vi "initiateProducts.vi"(0 "reference in":refnum<class "Project Panels.lvclass">, 5 "error in (no error)":errorcluster) -> (14 "reference out":refnum<class "Project Panels.lvclass">, 16 "tables":T1, 19 "error out":errorcluster)   [LabVIEW 2016, in "Project Panels.lvclass"]
uses:
  Project Panels.lvclass
  SYS/Devices Controller_llb/Devices Controller.lvclass
  APP/k4b2_class/k4b2.lvclass
  APP/rmr_class/rmr.lvclass
  APP/bodpod_class/bodpod.lvclass
  APP/cpet_class/cpet.lvclass
  APP/fitmate_class/fitmate.lvclass
  APP/peapod_class/peapod.lvclass
  APP/k5_class/k5.lvclass
  APP/bb-pft_class/bb-pft.lvclass
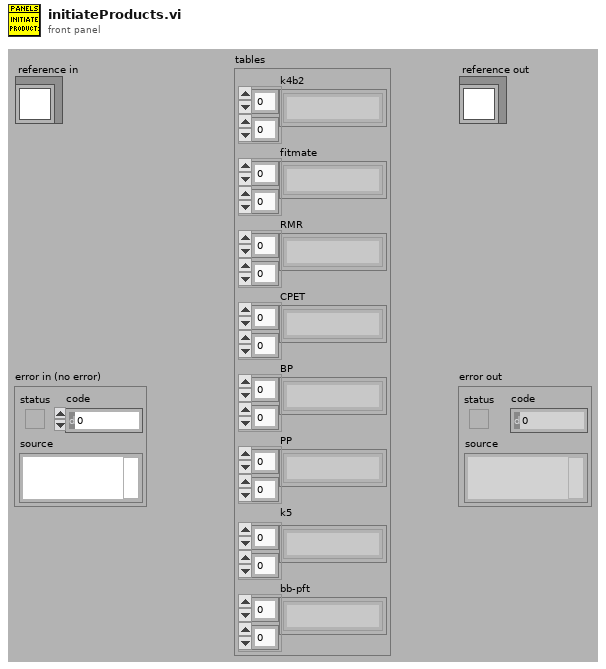
[diagram p1: front panel]
types:
  T1 = cluster{"k4b2":string[][], "fitmate":string[][], "RMR":string[][], "CPET":string[][], "BP":string[][], "PP":string[][], "k5":string[][], "bb-pft":string[][]}
  T2 = typedef "Project Panels.lvclass/ObjectAttributesRef.ctl" = refnum<data-value>
  T3 = typedef "Project Panels.lvclass/ObjectAttributes.ctl" = cluster{"MyAttribute":dbl, "device_controller_ref":refnum<class "Devices Controller.lvclass">, "file_controller_ref":refnum<class "File Controller.lvclass">, "item_controller_ref":refnum<class "Items Controller.lvclass">, "item_tables":cluster{"checkIN":string[][], "checkOUT":string[][], "storage":string[][]}, "quickbook_table":cluster{"notes":string[][]}, "notification_controller_ref":refnum<class "Notification Controller.lvclass">, "partstracking_controller_ref":refnum<class "PartsTracking Controller.lvclass">, "product_tables":cluster{"k4b2":string[][], "fitmate":string[][], "RMR":string[][], "CPET":string[][], "BP":string[][], "PP":string[][], "k5":string[][], "bb-pft":string[][]}, "rowsColour":u32[], "low_resolution?":bool, "run_python?":bool}
  T4 = cluster{"k4b2_refs":refnum<class "k4b2.lvclass">[], "rmr_refs":refnum<class "rmr.lvclass">[], "bod_pod_refs":refnum<class "bodpod.lvclass">[], "cpet_refs":refnum<class "cpet.lvclass">[], "fitmate_refs":refnum<class "fitmate.lvclass">[], "pea_pod_refs":refnum<class "peapod.lvclass">[], "k5_refs":refnum<class "k5.lvclass">[], "bb-pft_refs":refnum<class "bb-pft.lvclass">[]}
  T5 = typedef "Devices Controller.lvclass/deviceType.ctl" = enum16{"k5", "k4b2", "fitmate", "cpet", "rmr", "bodyBoxPft", "bp", "pp"}
  T6 = cluster{"deviceType":T5, "S/N":string, "SW":string, "Description":string, "Account":string, "System's Location":string, "End User":string, "Email":string, "City":string, "LastChange":string, "Service By":string, "Exp Date":string, "FollowUp Sent":string, "FollowUp Accepted":string, "Note":string}
  T7 = cluster{"deviceType":T5, "S/N":string, "SW":string, "Description":string, "Account":string, "System's Location":string, "End User":string, "Email":string, "City":string, "FollowUp Sent":string, "FollowUp Accepted":string, "Note":string}
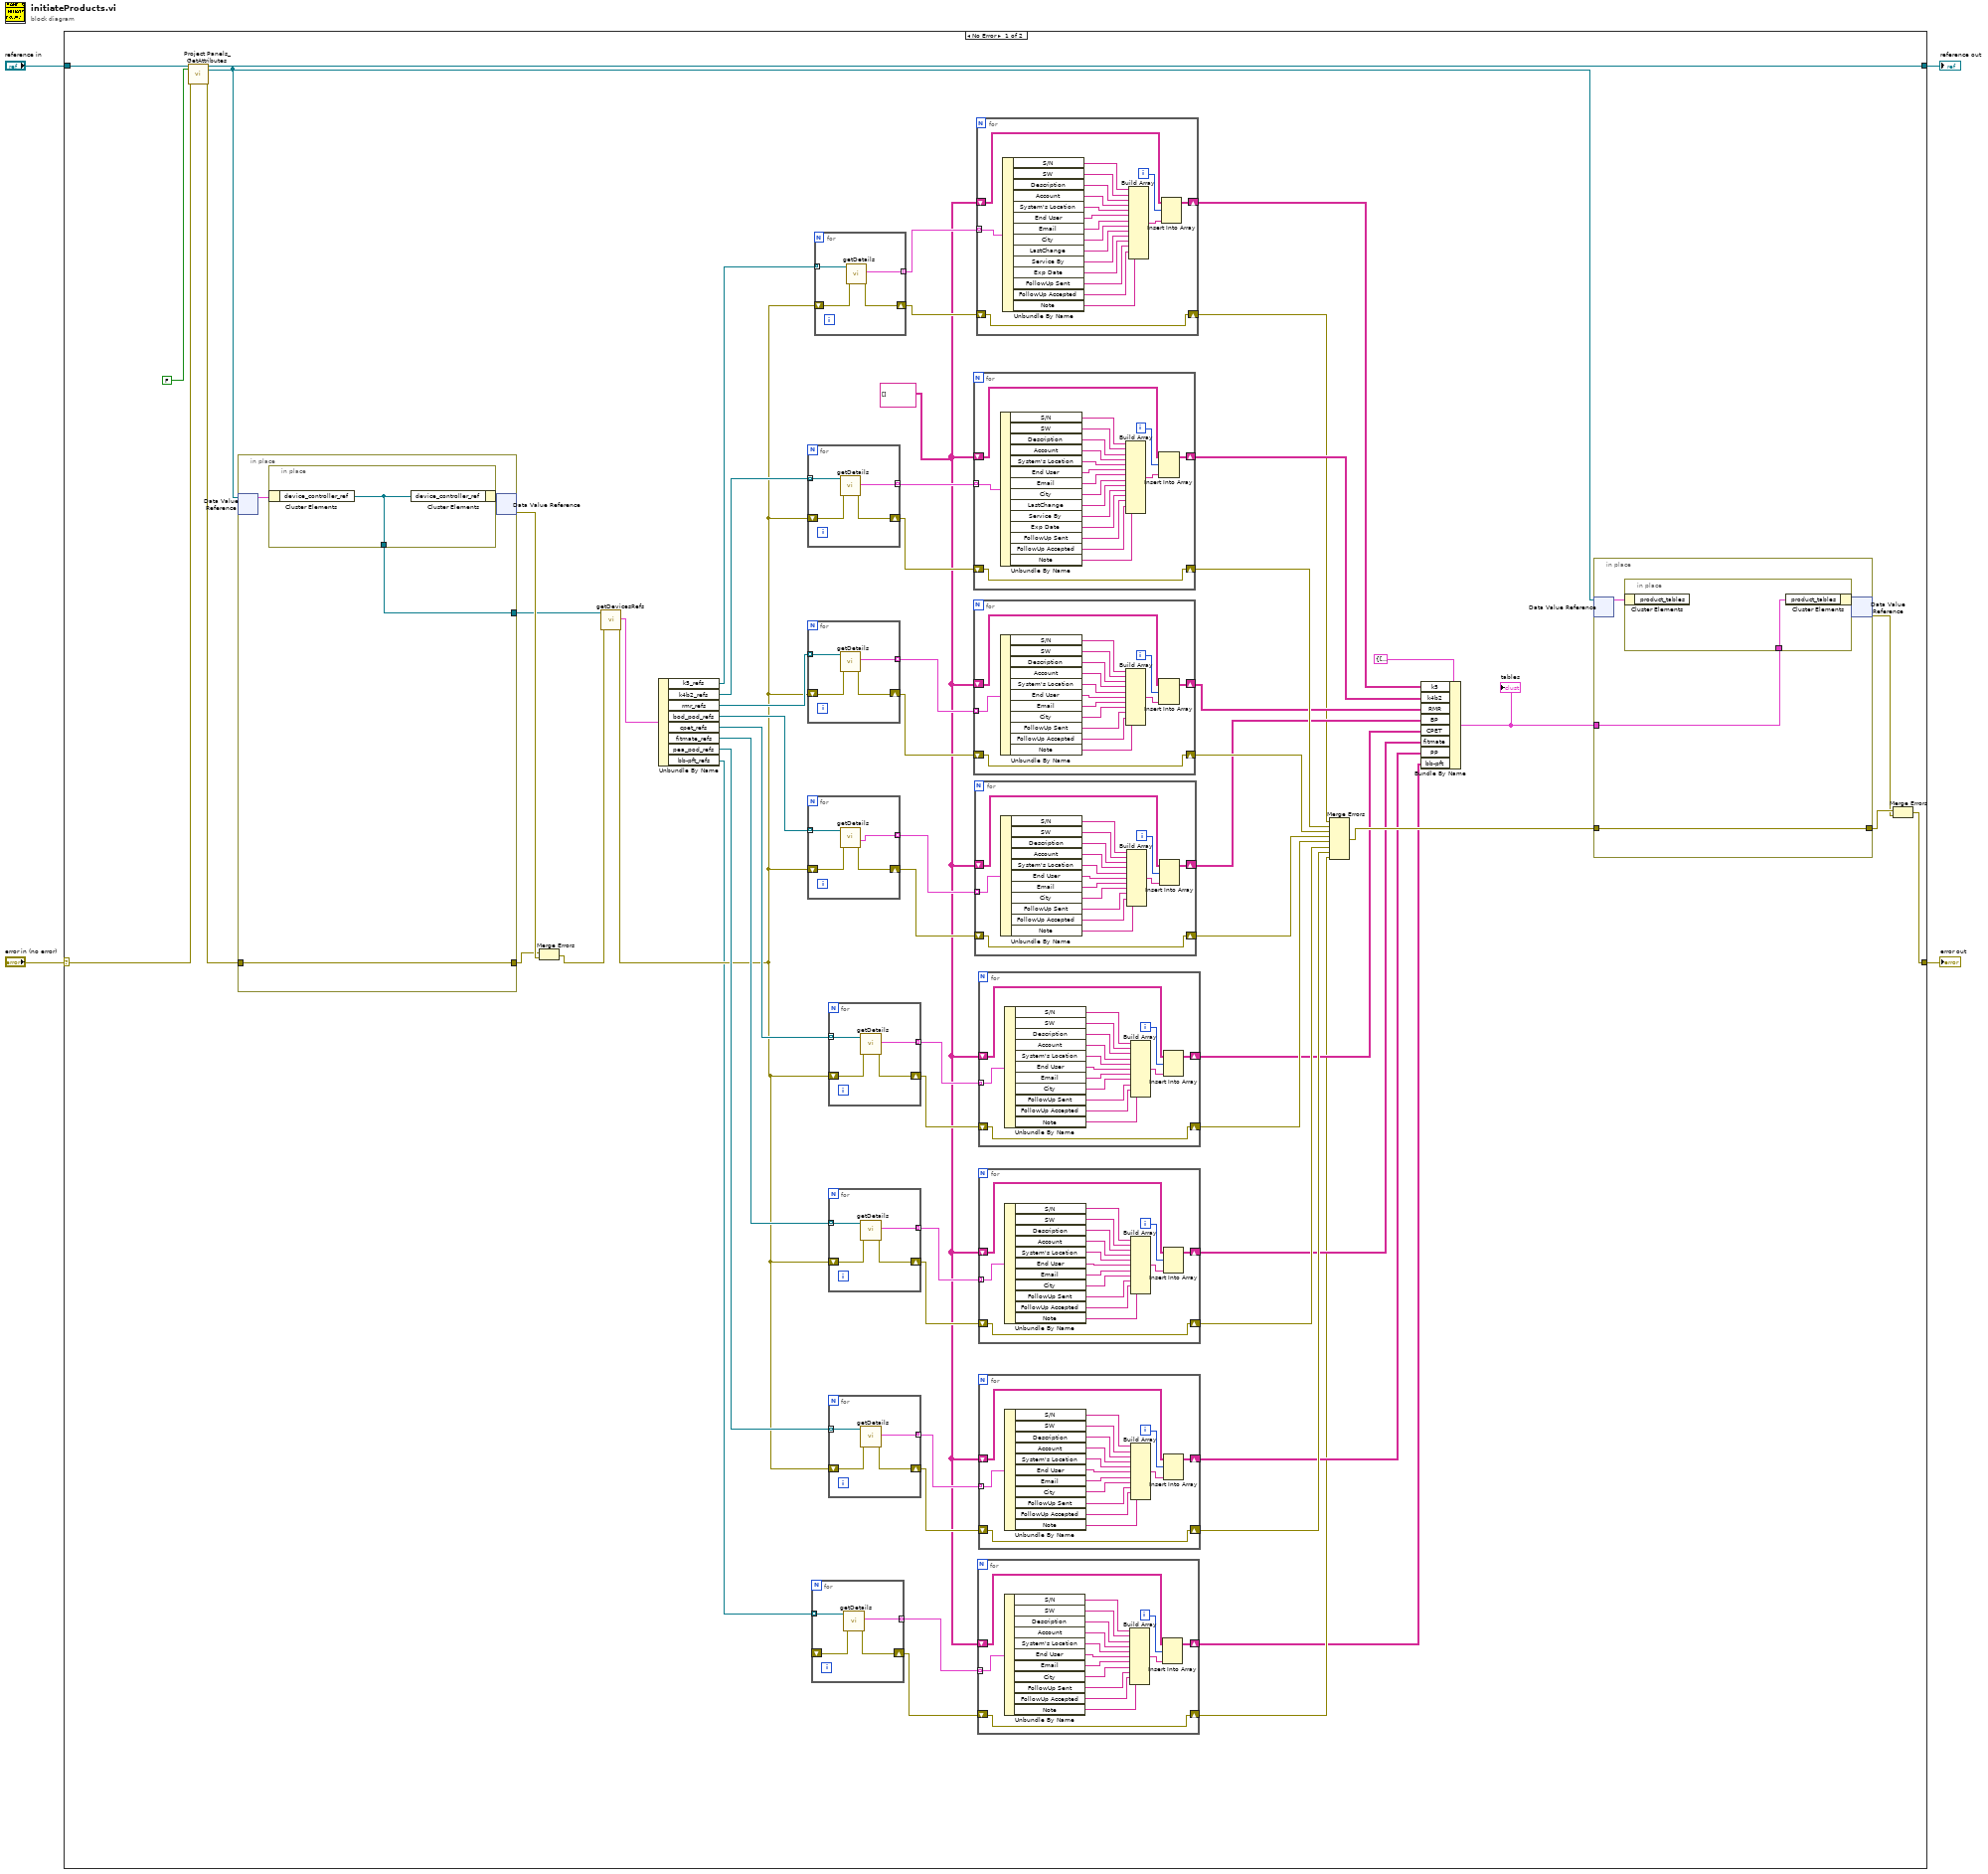
[diagram p0: block diagram]
diagram:
  n1 = case shown="No Error" "error in (no error)" {
    selector: "error in (no error)" -> [w20 w249]
    tunnel: [w21 w249] -> w3
    tunnel: [w58 w248] -> w1
    tunnel: "reference in" -> [w61 w248]
    frame No Error {
      w10 = string[][] [] ("Table Control")
      n2 = call "Project Panels_GetAttributes.vi"("reference in"=w61, "return data? (T)"=FALSE, "error in (no error)"=w20) -> ("reference out"=w58:refnum<class "Project Panels.lvclass">, "attributes ref"=w31:T2, "error out"=w59:errorcluster)  [unwired: 13 in, 1 out]
      n3 = in-place {
        in-place-border: w59 -> [w244]
        in-place-border: [w244] -> w62
        in-place-border: [w243] -> w19
        n4 = in-place-dvr #1(w31) -> (w245:T3)  [unwired: 1 out]
        n5 = in-place {
          in-place-border: [w247] -> w243
          n6 = in-place-cluster #2(w245) -> ("device_controller_ref"=w247:refnum<class "Devices Controller.lvclass">)
          n7 = in-place-cluster #2("device_controller_ref"=w247) -> (w246:T3)
        }
        n8 = in-place-dvr #1(w246) -> (w63:errorcluster)  [unwired: 1 out]
      }
      n9 = Merge Errors(w62, w63) -> (w56:errorcluster)
      n10 = call "getDevicesRefs.vi"("error in (no error)"=w56, "reference in"=w19) -> ("error out"=w14:errorcluster, "devices_refs"=w57:T4)  [unwired: 7 in, 1 out]
      n11 = Unbundle By Name(w57) -> ("k5_refs"=w15:refnum<class "k5.lvclass">[], "k4b2_refs"=w55:refnum<class "k4b2.lvclass">[], "rmr_refs"=w53:refnum<class "rmr.lvclass">[], "bod_pod_refs"=w51:refnum<class "bodpod.lvclass">[], "cpet_refs"=w47:refnum<class "cpet.lvclass">[], "fitmate_refs"=w44:refnum<class "fitmate.lvclass">[], "pea_pod_refs"=w41:refnum<class "peapod.lvclass">[], "bb-pft_refs"=w8:refnum<class "bb-pft.lvclass">[])
      n12 = for {
        shift-right: [w241] -> w17
        shift-left: w14 -> [w242]
        tunnel: [w240] -> w54 mode=indexing
        tunnel: w55 -> [w239] mode=indexing
        n13 = call "getDetails.vi"("error in (no error)"=w242, "reference in"=w239) -> ("error out"=w241:errorcluster, "details"=w240:T6)  [unwired: 7 in, 1 out]
      }
      n14 = for {
        shift-right: [w217] -> w52
        shift-left: w14 -> [w218]
        tunnel: [w216] -> w49 mode=indexing
        tunnel: w53 -> [w215] mode=indexing
        n15 = call "getDetails.vi"("error in (no error)"=w218, "reference in"=w215) -> ("error out"=w217:errorcluster, "details"=w216:T7)  [unwired: 7 in, 1 out]
      }
      n16 = for {
        shift-right: [w179] -> w48
        shift-left: w14 -> [w180]
        tunnel: [w177] -> w50 mode=indexing
        tunnel: w51 -> [w178] mode=indexing
        n17 = call "getDetails.vi"("error in (no error)"=w180, "reference in"=w178) -> ("error out"=w179:errorcluster, "details"=w177:T7)  [unwired: 7 in, 1 out]
      }
      n18 = for {
        shift-right: [w83] -> w11
        shift-left: _ -> [w84]
        tunnel: [w82] -> w9 mode=indexing
        tunnel: w8 -> [w81] mode=indexing
        n19 = call "getDetails.vi"("error in (no error)"=w84, "reference in"=w81) -> ("error out"=w83:errorcluster, "details"=w82:T7)  [unwired: 7 in, 1 out]
      }
      n20 = for {
        shift-right: [w87] -> w16
        shift-left: w14 -> [w88]
        tunnel: [w86] -> w13 mode=indexing
        tunnel: w15 -> [w85] mode=indexing
        n21 = call "getDetails.vi"("error in (no error)"=w88, "reference in"=w85) -> ("error out"=w87:errorcluster, "details"=w86:T6)  [unwired: 7 in, 1 out]
      }
      n22 = for {
        shift-right: [w158] -> w45
        shift-left: w14 -> [w159]
        tunnel: [w156] -> w46 mode=indexing
        tunnel: w47 -> [w157] mode=indexing
        n23 = call "getDetails.vi"("error in (no error)"=w159, "reference in"=w157) -> ("error out"=w158:errorcluster, "details"=w156:T7)  [unwired: 7 in, 1 out]
      }
      n24 = for {
        shift-right: [w137] -> w43
        shift-left: w14 -> [w138]
        tunnel: [w136] -> w42 mode=indexing
        tunnel: w44 -> [w135] mode=indexing
        n25 = call "getDetails.vi"("error in (no error)"=w138, "reference in"=w135) -> ("error out"=w137:errorcluster, "details"=w136:T7)  [unwired: 7 in, 1 out]
      }
      n26 = for {
        shift-right: [w116] -> w40
        shift-left: w14 -> [w117]
        tunnel: [w115] -> w39 mode=indexing
        tunnel: w41 -> [w114] mode=indexing
        n27 = call "getDetails.vi"("error in (no error)"=w117, "reference in"=w114) -> ("error out"=w116:errorcluster, "details"=w115:T7)  [unwired: 7 in, 1 out]
      }
      n28 = for {
        tunnel: w54 -> [w236] mode=indexing
        shift-right: [w237] -> w30
        shift-left: w10 -> [w238]
        shift-right: [w220] -> w37
        shift-left: w17 -> [w220]
        i -> [w233]
        n29 = Unbundle By Name(w236) -> ("S/N"=w235:string, "SW"=w232:string, "Description"=w231:string, "Account"=w230:string, "System's Location"=w229:string, "End User"=w228:string, "Email"=w227:string, "City"=w226:string, "LastChange"=w225:string, "Service By"=w224:string, "Exp Date"=w223:string, "FollowUp Sent"=w222:string, "FollowUp Accepted"=w221:string, "Note"=w219:string)
        n30 = Build Array(w235, w232, w231, w230, w229, w228, w227, w226, w225, w224, w223, w222, w221, w219) -> (w234:string[])
        n31 = Insert Into Array(array=w238, index (row)=w233, new element=w234) -> (w237:string[][])  [unwired: 1 in]
      }
      n32 = for {
        tunnel: w49 -> [w212] mode=indexing
        shift-right: [w213] -> w28
        shift-left: w10 -> [w214]
        shift-right: [w199] -> w36
        shift-left: w52 -> [w199]
        i -> [w209]
        n33 = Unbundle By Name(w212) -> ("S/N"=w211:string, "SW"=w208:string, "Description"=w207:string, "Account"=w206:string, "System's Location"=w205:string, "End User"=w204:string, "Email"=w203:string, "City"=w202:string, "FollowUp Sent"=w201:string, "FollowUp Accepted"=w200:string, "Note"=w198:string)
        n34 = Build Array(w211, w208, w207, w206, w205, w204, w203, w202, w201, w200, w198) -> (w210:string[])
        n35 = Insert Into Array(array=w214, index (row)=w209, new element=w210) -> (w213:string[][])  [unwired: 1 in]
      }
      n36 = for {
        tunnel: w50 -> [w195] mode=indexing
        shift-right: [w196] -> w27
        shift-left: w10 -> [w197]
        shift-right: [w183] -> w35
        shift-left: w48 -> [w183]
        i -> [w193]
        n37 = Unbundle By Name(w195) -> ("S/N"=w194:string, "SW"=w192:string, "Description"=w191:string, "Account"=w190:string, "System's Location"=w189:string, "End User"=w188:string, "Email"=w187:string, "City"=w186:string, "FollowUp Sent"=w185:string, "FollowUp Accepted"=w184:string, "Note"=w181:string)
        n38 = Build Array(w194, w192, w191, w190, w189, w188, w187, w186, w185, w184, w181) -> (w182:string[])
        n39 = Insert Into Array(array=w197, index (row)=w193, new element=w182) -> (w196:string[][])  [unwired: 1 in]
      }
      n40 = for {
        tunnel: w13 -> [w106] mode=indexing
        shift-right: [w107] -> w12
        shift-left: w10 -> [w108]
        shift-right: [w90] -> w7
        shift-left: w16 -> [w90]
        i -> [w103]
        n41 = Unbundle By Name(w106) -> ("S/N"=w105:string, "SW"=w102:string, "Description"=w101:string, "Account"=w100:string, "System's Location"=w99:string, "End User"=w98:string, "Email"=w97:string, "City"=w96:string, "LastChange"=w95:string, "Service By"=w94:string, "Exp Date"=w93:string, "FollowUp Sent"=w92:string, "FollowUp Accepted"=w91:string, "Note"=w89:string)
        n42 = Build Array(w105, w102, w101, w100, w99, w98, w97, w96, w95, w94, w93, w92, w91, w89) -> (w104:string[])
        n43 = Insert Into Array(array=w108, index (row)=w103, new element=w104) -> (w107:string[][])  [unwired: 1 in]
      }
      n44 = for {
        tunnel: w9 -> [w78] mode=indexing
        shift-right: [w79] -> w5
        shift-left: w10 -> [w80]
        shift-right: [w65] -> w6
        shift-left: w11 -> [w65]
        i -> [w75]
        n45 = Unbundle By Name(w78) -> ("S/N"=w77:string, "SW"=w74:string, "Description"=w73:string, "Account"=w72:string, "System's Location"=w71:string, "End User"=w70:string, "Email"=w69:string, "City"=w68:string, "FollowUp Sent"=w67:string, "FollowUp Accepted"=w66:string, "Note"=w64:string)
        n46 = Build Array(w77, w74, w73, w72, w71, w70, w69, w68, w67, w66, w64) -> (w76:string[])
        n47 = Insert Into Array(array=w80, index (row)=w75, new element=w76) -> (w79:string[][])  [unwired: 1 in]
      }
      n48 = for {
        tunnel: w46 -> [w174] mode=indexing
        shift-right: [w175] -> w26
        shift-left: w10 -> [w176]
        shift-right: [w162] -> w34
        shift-left: w45 -> [w162]
        i -> [w172]
        n49 = Unbundle By Name(w174) -> ("S/N"=w173:string, "SW"=w171:string, "Description"=w170:string, "Account"=w169:string, "System's Location"=w168:string, "End User"=w167:string, "Email"=w166:string, "City"=w165:string, "FollowUp Sent"=w164:string, "FollowUp Accepted"=w163:string, "Note"=w160:string)
        n50 = Build Array(w173, w171, w170, w169, w168, w167, w166, w165, w164, w163, w160) -> (w161:string[])
        n51 = Insert Into Array(array=w176, index (row)=w172, new element=w161) -> (w175:string[][])  [unwired: 1 in]
      }
      n52 = for {
        tunnel: w42 -> [w153] mode=indexing
        shift-right: [w154] -> w25
        shift-left: w10 -> [w155]
        shift-right: [w141] -> w33
        shift-left: w43 -> [w141]
        i -> [w151]
        n53 = Unbundle By Name(w153) -> ("S/N"=w152:string, "SW"=w150:string, "Description"=w149:string, "Account"=w148:string, "System's Location"=w147:string, "End User"=w146:string, "Email"=w145:string, "City"=w144:string, "FollowUp Sent"=w143:string, "FollowUp Accepted"=w142:string, "Note"=w139:string)
        n54 = Build Array(w152, w150, w149, w148, w147, w146, w145, w144, w143, w142, w139) -> (w140:string[])
        n55 = Insert Into Array(array=w155, index (row)=w151, new element=w140) -> (w154:string[][])  [unwired: 1 in]
      }
      n56 = for {
        tunnel: w39 -> [w132] mode=indexing
        shift-right: [w133] -> w24
        shift-left: w10 -> [w134]
        shift-right: [w120] -> w32
        shift-left: w40 -> [w120]
        i -> [w130]
        n57 = Unbundle By Name(w132) -> ("S/N"=w131:string, "SW"=w129:string, "Description"=w128:string, "Account"=w127:string, "System's Location"=w126:string, "End User"=w125:string, "Email"=w124:string, "City"=w123:string, "FollowUp Sent"=w122:string, "FollowUp Accepted"=w121:string, "Note"=w118:string)
        n58 = Build Array(w131, w129, w128, w127, w126, w125, w124, w123, w122, w121, w118) -> (w119:string[])
        n59 = Insert Into Array(array=w134, index (row)=w130, new element=w119) -> (w133:string[][])  [unwired: 1 in]
      }
      n60 = Merge Errors(w7, w37, w36, w35, w34, w33, w32, w6) -> (w38:errorcluster)
      n61 = Bundle By Name(cluster=T1 {"k4b2"=[], "fitmate"=[], "RMR"=[], "CPET"=[], "BP"=[], "PP"=[], "k5"=[], "bb-pft"=[]} ("tables 2"), "k5"=w12, "k4b2"=w30, "RMR"=w28, "BP"=w27, "CPET"=w26, "fitmate"=w25, "PP"=w24, "bb-pft"=w5) -> (w29:T1)
      "tables" <- w29
      n62 = in-place {
        in-place-border: w38 -> [w110]
        in-place-border: [w110] -> w23
        in-place-border: w29 -> [w109]
        n63 = in-place-dvr #3(w31) -> (w111:T3)  [unwired: 1 out]
        n64 = in-place {
          in-place-border: w109 -> [w113]
          n65 = in-place-cluster #4(w111) -> ()  [unwired: 1 out]
          n66 = in-place-cluster #4("product_tables"=w113) -> (w112:T3)
        }
        n67 = in-place-dvr #3(w112) -> (w22:errorcluster)  [unwired: 1 out]
      }
      n68 = Merge Errors(w23, w22) -> (w21:errorcluster)
    }
    frame Error {
    }
  }
  "error out" <- w3
  "reference out" <- w1
